vi "Check for Mail.vi"(4 "error in":errorcluster, 7 "connection ID in":refnum<k5>) -> (0 "error out":errorcluster, 1 "LIST response":string="\r\n", 2 "# messages":i32 min=0, 3 "connection ID out":refnum<k5>)   [LabVIEW 2012]
doc: "This mid-level VI queries a POP mail server to see if there are any new messages waiting to be read, returning the number of messages found and the actual query response from the POP server.\n\nIt is assumed that a connection with the mail server has already been established prior to calling this VI."
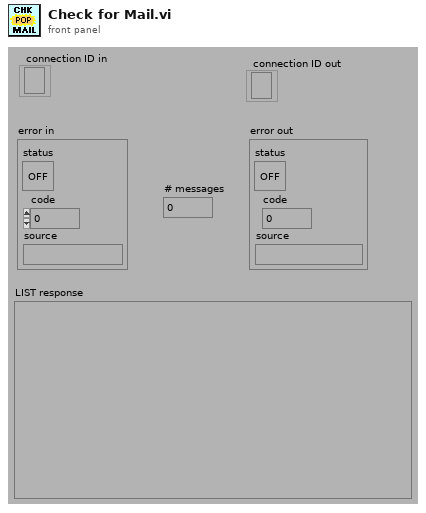
[diagram p1: front panel]
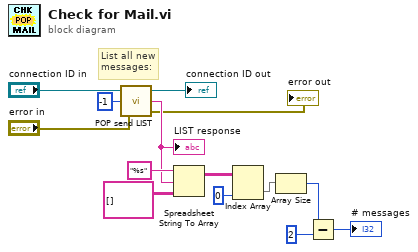
[diagram p0: block diagram]
diagram:
  # "List all new\nmessages:"
  n1 = call "POP send LIST.vi"("error in"="error in", "MSG number"=-1, "connection ID in"="connection ID in") -> ("error out"=→"error out":errorcluster, "LIST response"=w3:string, "connection ID out"=→"connection ID out":refnum<k5>)
  "LIST response" <- w3
  n2 = Spreadsheet String To Array(format string="%s", spreadsheet string=w3, array type (2D Dbl)=string[][] []) -> (array=w12:string[][])  [unwired: 1 in]
  n3 = Index Array(array=w12, index (col)=0) -> (element=w9:string[])  [unwired: 1 in]
  n4 = Array Size(array=w9) -> (size(s)=w8:i32)
  n5 = Subtract(x=w8, y=2) -> (x-y=→"# messages":i32)
